vi "UI_AutoRefresh_Do.vi"(8 "error in (no error)":errorcluster, 9 "Parameters":T1={"Write TipStrips with details (T)"=TRUE, "Write Captions with UserLabels (T)"=TRUE, "Mode (ind only)"=enum."Indicators only", "Enable nested stream (T)"=TRUE}, 10 "Databox_sealed":refnum<class "Databox_sealed.lvclass">, 11 "UI_Actor in":refnum<class "UI_Actor.lvclass">) -> (0 "error out":errorcluster, 3 "UI_Actor out":refnum<class "UI_Actor.lvclass">)   [LabVIEW 2020, in "UI_Actor.lvlib" / "UI_Actor.lvclass"]
doc: "Enable nested stream : Permet le routage de la databox vers les nested UIA de l'acteur. On peut couper ce ruissellement si les nested n'ont pas besoin de databox pour optimiser le programme."
uses:
  UI_Actor.lvclass
  UI_Actor Messages/UI_AutoRefresh_Do Msg/UI_AutoRefresh_Do Msg.lvclass
  support/Databox.lvlibp/Databox_sealed/Databox_sealed.lvclass
  support/Actor Framework.lvlibp/1abvi3w/vi.lib/ActorFramework/Message Enqueuer/Message Enqueuer.lvclass
  support/Actor Framework.lvlibp/1abvi3w/vi.lib/ActorFramework/Message/Message.lvclass
  ctl_AR_Mode.ctl
  ctl_AR_Parameters.ctl
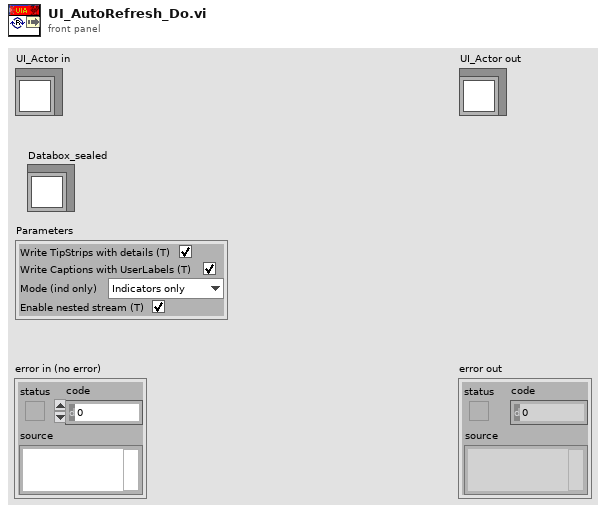
[diagram p1: front panel]
types:
  T1 = typedef "UI_Actor.lvlib/UI_Actor.lvclass/ctl_AR_Parameters.ctl" = cluster{"Write TipStrips with details (T)":bool, "Write Captions with UserLabels (T)":bool, "Mode (ind only)":T2, "Enable nested stream (T)":bool}
  T2 = typedef "UI_Actor.lvlib/UI_Actor.lvclass/ctl_AR_Mode.ctl" = enum16{"Controls only", "Indicators only", "All"}
  T3 = typedef "UI_Actor.lvlib/UI_Actor.lvclass/ctl_AR_Elmt.ctl" = cluster{"AR by Index":bool, "Ref":refnum<vi>, "Index":i32, "Class ID":u32, "Sourcer":string, "SysLab":string}
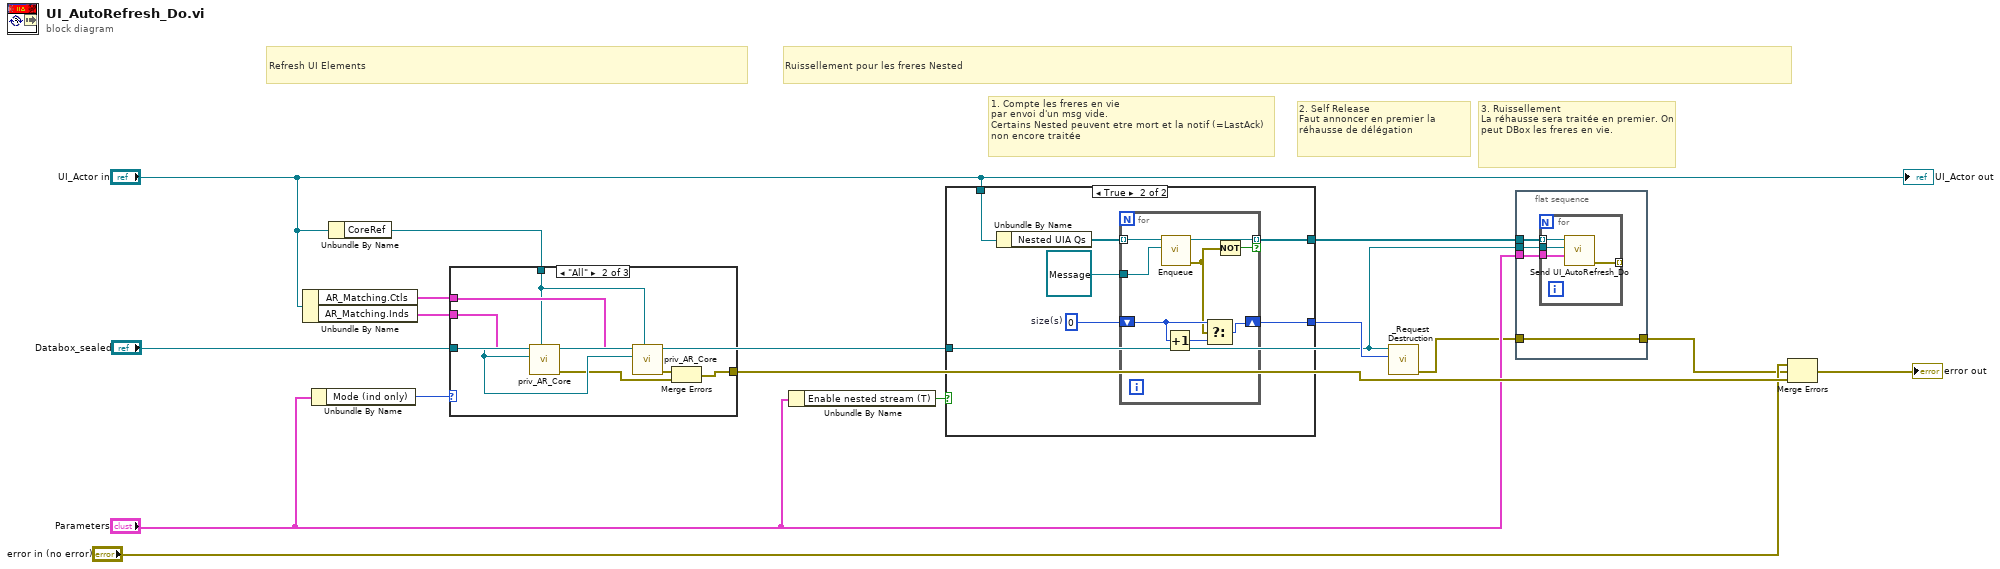
[diagram p0: block diagram]
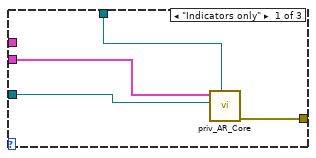
[diagram p3: hidden frame]
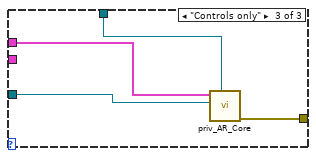
[diagram p4: hidden frame]
diagram:
  # "3. Ruissellement\nLa réhausse sera traitée en premier. On peut DBox les freres en vie."
  # "1. Compte les freres en vie\npar envoi d'un msg vide.\nCertains Nested peuvent etre mort et la notif (=LastAck) non encore traitée"
  # "2. Self Release\nFaut annoncer en premier la réhausse de délégation"
  # "Ruissellement pour les freres Nested"
  # "Refresh UI Elements"
  n1 = Unbundle By Name("UI_Actor in") -> ("AR_Matching.Ctls"=w12:T3[], "AR_Matching.Inds"=w13:T3[])
  n2 = Unbundle By Name("Parameters") -> ("Mode (ind only)"=w10:T2)
  n3 = Unbundle By Name("UI_Actor in") -> ("CoreRef"=w9:refnum<vi>)
  n4 = case shown="\"All\"" w10 {
    tunnel: "Databox_sealed" -> [w19 w24 w30]
    tunnel: w13 -> [w18 w26 _]
    tunnel: w12 -> [_ w25 w29]
    tunnel: [w17 w22 w28] -> w8
    tunnel: w9 -> [w16 w20 w27]
    frame "Indicators only" {
      n5 = call "priv_AR_Core.vi"("CoreRef"=w16, "Databox_sealed"=w19, "AR_Matching"=w18) -> ("error out"=w17:errorcluster)  [unwired: 8 in]
    }
    frame "All" {
      n6 = call "priv_AR_Core.vi"("CoreRef"=w20, "Databox_sealed"=w24, "AR_Matching"=w26) -> ("error out"=w21:errorcluster)  [unwired: 8 in]
      n7 = call "priv_AR_Core.vi"("CoreRef"=w20, "Databox_sealed"=w24, "AR_Matching"=w25) -> ("error out"=w23:errorcluster)  [unwired: 8 in]
      n8 = Merge Errors(w23, w21) -> (w22:errorcluster)
    }
    frame "Controls only" {
      n9 = call "priv_AR_Core.vi"("CoreRef"=w27, "Databox_sealed"=w30, "AR_Matching"=w29) -> ("error out"=w28:errorcluster)  [unwired: 8 in]
    }
  }
  n10 = Unbundle By Name("Parameters") -> ("Enable nested stream (T)"=w6:bool)
  n11 = case shown="True" w6 {
    tunnel: [_ w35] -> w11
    tunnel: "Databox_sealed" -> [_ _]
    tunnel: "UI_Actor in" -> [_ w34]
    tunnel: [_ w31] -> w5
    frame False {
    }
    frame True {
      w33 = 0  # size(s)
      n12 = Unbundle By Name(w34) -> ("Nested UIA Qs"=w36:refnum<class "Message Enqueuer.lvclass">[])
      n13 = for {
        tunnel: w36 -> [w41] mode=indexing
        shift-right: [w43] -> w35
        shift-left: w33 -> [w42]
        tunnel: refnum<class "Message.lvclass"> refnum ("Message") -> [w40]
        tunnel: [w39] -> w31 mode=indexing if=w37
        n14 = call "Enqueue.vi"("Message"=w40, "Message Enqueuer in"=w41) -> ("error out"=w38:errorcluster, "Message Enqueuer out"=w39:refnum<class "Message Enqueuer.lvclass">)  [unwired: 8 in]
        n15 = Increment(x=w42) -> (x+1=w44:i32)
        n16 = Select(t=w42, s=w38, f=w44) -> (s? t:f=w43:i32)
        n17 = Not(x=w38) -> (.not. x?=w37:bool)
      }
    }
  }
  n18 = call "_Request Destruction.vi"("Additionnal delegations (0)"=w11, "Databox_sealed in"="Databox_sealed") -> ("error out"=w2:errorcluster)  [unwired: 9 in]
  n19 = flat-sequence {
    tunnel: w5 -> [w48]
    tunnel: "Databox_sealed" -> [w47]
    tunnel: "Parameters" -> [w46]
    tunnel: [w45] -> w1
    tunnel: w2 -> [w45]
    frame #0 {
      n20 = for {
        tunnel: w48 -> [w52] mode=indexing
        tunnel: w46 -> [w51]
        tunnel: w47 -> [w50]
        tunnel: [w49] -> _ mode=indexing
        n21 = call "Send UI_AutoRefresh_Do.vi"("Parameters"=w51, "Databox_sealed"=w50, "Message Enqueuer"=w52) -> ("error out"=w49:errorcluster)  [unwired: 7 in, 1 out]
      }
    }
  }
  n22 = Merge Errors("error in (no error)", w1, w8) -> (→"error out":errorcluster)
  "UI_Actor out" <- "UI_Actor in"
